vi "MakeDataFileNames_theirs.vi"(4 "seconds since 1904 (default 0 = now)":u32, 6 "File Prefix":string="s", 7 "File format":T1, 8 "error in (no error)":errorcluster, 9 "Interactive":bool=TRUE, 10 "Generate Index":bool=TRUE, 11 "Root Data Folder":path=path "C:/Data") -> (0 "error out":errorcluster, 2 "Settings File Path":path, 3 "Data File  Path":path)   [LabVIEW 2024]
uses:
  Controls/File formats.ctl
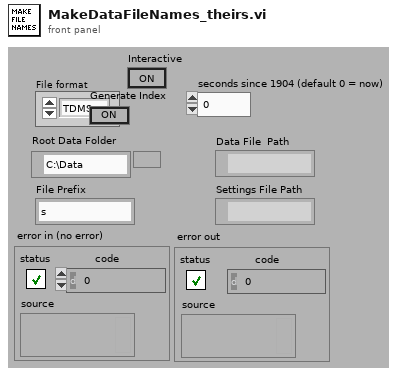
[diagram p1: front panel]
types:
  T1 = typedef "File formats.ctl" = enum16{"TDMS", "ASCII", "BINARY"}
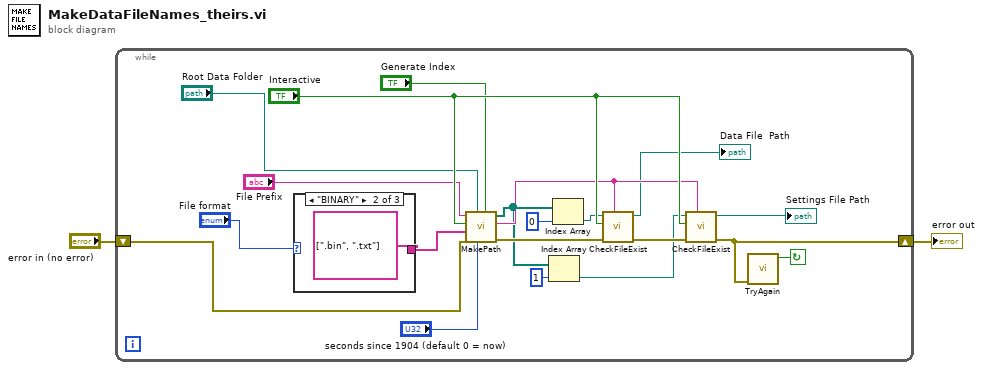
[diagram p0: block diagram]
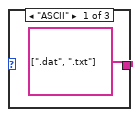
[diagram p2: hidden frame]
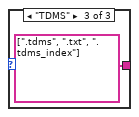
[diagram p3: hidden frame]
diagram:
  n1 = while {
    shift-right: [w21] -> w2
    shift-left: "error in (no error)" -> [w10]
    stop <- w20 continue-if-true
    n2 = case shown="\"BINARY\"" "File format" {
      tunnel: [string[] [".dat", ".txt"] string[] [".bin", ".txt"] string[] [".tdms", ".txt", ".tdms_index"]] -> w17
      frame "ASCII" {
      }
      frame "BINARY" {
      }
      frame "TDMS" {
      }
    }
    n3 = call "MakePath.vi"("Generate Index"="Generate Index", "seconds since 1904 (default 0 = now)"="seconds since 1904 (default 0 = now)", "Root Data Folder"="Root Data Folder", "Error In"=w10, "Extentions"=w17, "Interactive"="Interactive", "File Prefix"="File Prefix") -> ("Error Out"=w19:errorcluster, "format string"=w16:string, "Paths out"=w11:path[])  [unwired: 2 in]
    n4 = Index Array(array=w11, index=1) -> (element=w12:path)
    n5 = Index Array(array=w11, index=0) -> (element=w13:path)
    n6 = call "CheckFileExist.vi"("format string"=w16, "error in (no error) 2"=w19, "Interactive"="Interactive", "File in"=w13) -> ("error out"=w18:errorcluster, "File out"=→"Data File  Path":path)  [unwired: 6 out]
    n7 = call "CheckFileExist.vi"("format string"=w16, "error in (no error) 2"=w18, "Interactive"="Interactive", "File in"=w12) -> ("error out"=w21:errorcluster, "File out"=→"Settings File Path":path)  [unwired: 6 out]
    n8 = call "TryAgain.vi"("error in (no error)"=w21) -> ("Try again"=w20:bool)  [unwired: 6 out]
  }
  "error out" <- w2
